vi "Send_UIDisableCtrlArray.vi"(8 "error in":errorcluster, 9 "Disabled":T1(array[ring]), 10 "Control Label":string[](array[string]), 11 "Queue in":refnum<queue>) -> (0 "error out":errorcluster)   [LabVIEW 2018, in "UI_Library.lvlib"]
uses:
  UI_Library.lvlib
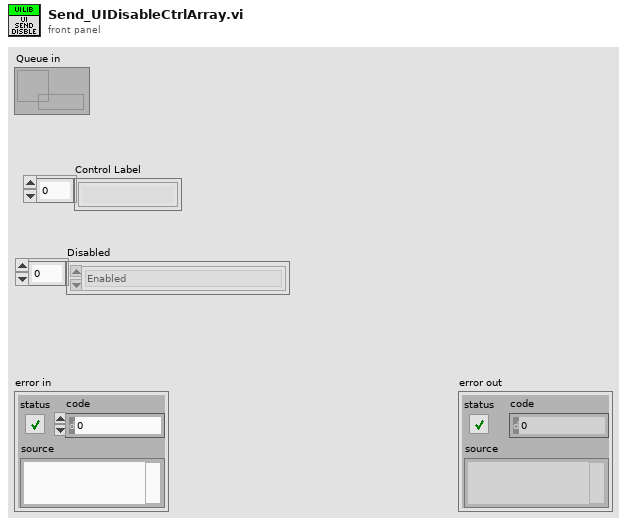
[diagram p1: front panel]
types:
  T1 = enum8{"Enabled", "Disabled", "Disabled and Grayed Out"}[]
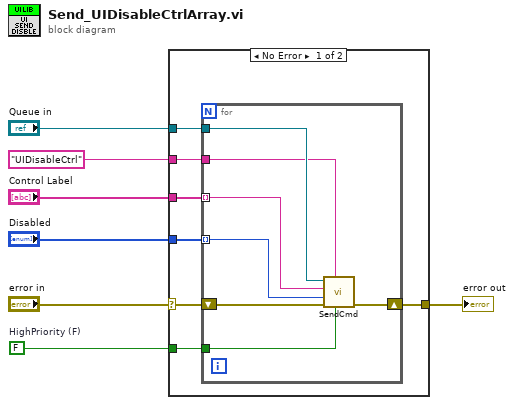
[diagram p0: block diagram]
diagram:
  w5 = FALSE  # HighPriority (F)
  n1 = case shown="No Error" "error in" {
    selector: "error in" -> [w13 w22]
    tunnel: "Queue in" -> [w14 _]
    tunnel: "Control Label" -> [w10 _]
    tunnel: "Disabled" -> [w9 _]
    tunnel: "UIDisableCtrl" ("UICmd") -> [w11 _]
    tunnel: w5 -> [w8 _]
    tunnel: [w12 w22] -> w7
    frame No Error {
      n2 = for {
        tunnel: w14 -> [w21]
        tunnel: w11 -> [w18]
        tunnel: w10 -> [w17] mode=indexing
        tunnel: w9 -> [w16] mode=indexing
        tunnel: w8 -> [w15]
        shift-right: [w19] -> w12
        shift-left: w13 -> [w20]
        n3 = call "SendCmd.vi"("HighPriority (F)"=w15, "UICmd"=w18, "error in"=w20, "Control Data"=w16, "Control Label"=w17, "Queue in"=w21) -> ("error out"=w19:errorcluster)  [unwired: 5 in]
      }
    }
    frame Error {
    }
  }
  "error out" <- w7
